vi "Data Queue manager.vi"(5 "queue size":i32, 7 "Action":T1=enum."Enqueue", 8 "error in":errorcluster, 11 "Buffer":sgl[](array[numeric])) -> (0 "error out":errorcluster, 2 "Empty?":bool, 3 "data out":sgl[](array[numeric]))   [LabVIEW 2018]
uses:
  Controls/Queue Manager Actions.ctl
  Controls/QueueNames.ctl
  Controls/MessagePacket.ctl
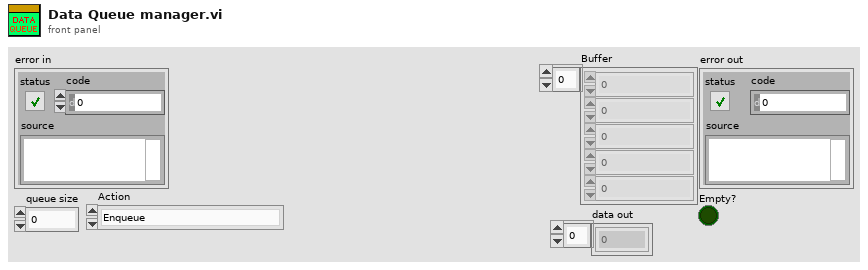
[diagram p1: front panel]
types:
  T1 = typedef "Queue Manager Actions.ctl" = enum16{"Init", "Enqueue", "Enqueue All", "Preview Queue", "Dequeue", "Get Status", "Flush Queue", "Flush All Queues", "Release All Queues", "Release Queue", "Enqueue at Opposite End"}
  T2 = typedef "MessagePacket.ctl" = cluster{"Message":string, "Parameter":variant}
  T3 = typedef "QueueNames.ctl" = enum16{"Main GUI", "Main Scan Processor", "Main Processing", "Main Saving", "Main Display", "Main Table Stage GUI", "Main Table Stage Proc.", "Scan Engine", "Vibratome GUI", "Vibratome Processor", "Slice Engine"}
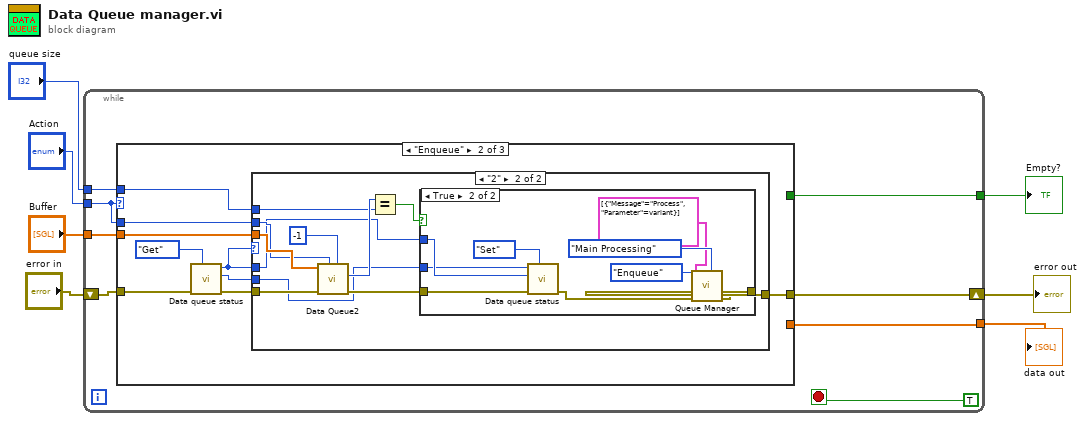
[diagram p0: block diagram]
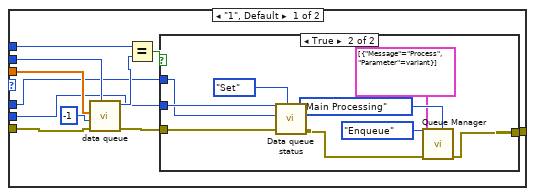
[diagram p3: hidden frame]
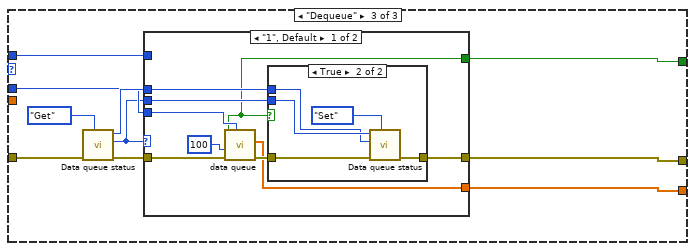
[diagram p6: hidden frame]
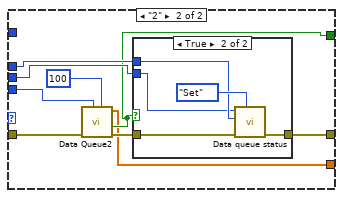
[diagram p8: hidden frame]
diagram:
  n1 = while {
    tunnel: "Buffer" -> [w15]
    tunnel: "Action" -> [w14]
    tunnel: "queue size" -> [w12]
    shift-right: [w11] -> w3
    shift-left: "error in" -> [w13]
    tunnel: [w9] -> w2
    tunnel: [w8] -> w1
    stop <- TRUE stop-if-true
    n2 = case shown="\"Enqueue\"" w14 {
      tunnel: w15 -> [_ w25 _]
      tunnel: w13 -> [w16 w22 w74]
      tunnel: w14 -> [_ w24 w73]
      tunnel: w12 -> [_ w20 w72]
      tunnel: [w16 w17 w71] -> w11
      tunnel: [_ _ w69] -> w9
      tunnel: [_ _ w68] -> w8
      frame "Init", Default {
      }
      frame "Enqueue" {
        n3 = call "Data queue status.vi"("action"=enum16{"Init", "Get", "Set"}."Get", "error in"=w22) -> ("error out"=w21:errorcluster, "dequeue channel"=w18:enum16{"1", "2"}, "enqueue channel"=w19:enum16{"1", "2"})  [unwired: 7 in]
        n4 = case shown="\"2\"" w19 {
          tunnel: w25 -> [w32 w56]
          tunnel: w24 -> [w31 w55]
          tunnel: w21 -> [w35 w57]
          tunnel: w20 -> [w29 w52]
          tunnel: w19 -> [w27 w49]
          tunnel: w18 -> [w28 w48]
          tunnel: [w26 w47] -> w17
          frame "1", Default {
            n5 = call "data queue.vi"("Action"=w31, "error in (no error)"=w35, "timeout in ms (-1)"=-1, "data in"=w32) -> ("error out"=w34:errorcluster, "# elements in queue"=w30:i32)  [unwired: 4 in, 2 out]
            n6 = Equal?(x=w29, y=w30) -> (x = y?=w36:bool)
            n7 = case shown="True" w36 {
              tunnel: [w37 w39] -> w26
              tunnel: w34 -> [w37 w45]
              tunnel: w28 -> [_ w44]
              tunnel: w27 -> [_ w43]
              frame False {
              }
              frame True {
                n8 = call "Data queue status.vi"("action"=enum16{"Init", "Get", "Set"}."Set", "error in"=w45, "dequeue channel"=w43, "enqueue channel"=w44) -> ("error out"=w40:errorcluster)  [unwired: 5 in, 2 out]
                n9 = call "Queue Manager.vi"("Queue Name"=QueueNames."Main Processing", "Action"=Queue_Manager_Actions."Enqueue", "Error In"=w40, "Message Packet Array"=T2[] [{"Message"="Process", "Parameter"=variant}]) -> ("Error Out"=w39:errorcluster)  [unwired: 3 in, 4 out]
              }
            }
          }
          frame "2" {
            n10 = call "Data Queue2.vi"("timeout in ms (-1)"=-1, "Action"=w55, "error in (no error)"=w57, "data in"=w56) -> ("error out"=w50:errorcluster, "# elements in queue"=w53:i32)  [unwired: 4 in, 2 out]
            n11 = Equal?(x=w53, y=w52) -> (x = y?=w51:bool)
            n12 = case shown="True" w51 {
              tunnel: w50 -> [w58 w66]
              tunnel: w49 -> [_ w65]
              tunnel: w48 -> [_ w64]
              tunnel: [w58 w60] -> w47
              frame False {
              }
              frame True {
                n13 = call "Data queue status.vi"("action"=enum16{"Init", "Get", "Set"}."Set", "error in"=w66, "dequeue channel"=w65, "enqueue channel"=w64) -> ("error out"=w61:errorcluster)  [unwired: 5 in, 2 out]
                n14 = call "Queue Manager.vi"("Queue Name"=QueueNames."Main Processing", "Action"=Queue_Manager_Actions."Enqueue", "Error In"=w61, "Message Packet Array"=T2[] [{"Message"="Process", "Parameter"=variant}]) -> ("Error Out"=w60:errorcluster)  [unwired: 3 in, 4 out]
              }
            }
          }
        }
      }
      frame "Dequeue" {
        n15 = call "Data queue status.vi"("action"=enum16{"Init", "Get", "Set"}."Get", "error in"=w74) -> ("error out"=w76:errorcluster, "dequeue channel"=w70:enum16{"1", "2"}, "enqueue channel"=w75:enum16{"1", "2"})  [unwired: 7 in]
        n16 = case shown="\"1\", Default" w70 {
          tunnel: w73 -> [w83 w100]
          tunnel: w76 -> [w86 w101]
          tunnel: w72 -> [_ _]
          tunnel: w75 -> [w81 w97]
          tunnel: w70 -> [w82 w96]
          tunnel: [w80 w95] -> w71
          tunnel: [w79 w94] -> w69
          tunnel: [w78 w93] -> w68
          frame "1", Default {
            n17 = call "data queue.vi"("Action"=w83, "error in (no error)"=w86, "timeout in ms (-1)"=100) -> ("error out"=w85:errorcluster, "data out"=w78:sgl[], "Empty?"=w79:bool)  [unwired: 5 in, 1 out]
            n18 = case shown="True" w79 {
              tunnel: [w87 w91] -> w80
              tunnel: w85 -> [w87 w90]
              tunnel: w82 -> [_ w89]
              tunnel: w81 -> [_ w88]
              frame False {
              }
              frame True {
                n19 = call "Data queue status.vi"("action"=enum16{"Init", "Get", "Set"}."Set", "error in"=w90, "dequeue channel"=w88, "enqueue channel"=w89) -> ("error out"=w91:errorcluster)  [unwired: 5 in, 2 out]
              }
            }
          }
          frame "2" {
            n20 = call "Data Queue2.vi"("timeout in ms (-1)"=100, "Action"=w100, "error in (no error)"=w101) -> ("error out"=w98:errorcluster, "Empty?"=w94:bool, "data out"=w93:sgl[])  [unwired: 5 in, 1 out]
            n21 = case shown="True" w94 {
              tunnel: w98 -> [w102 w106]
              tunnel: w97 -> [_ w105]
              tunnel: w96 -> [_ w104]
              tunnel: [w102 w103] -> w95
              frame False {
              }
              frame True {
                n22 = call "Data queue status.vi"("action"=enum16{"Init", "Get", "Set"}."Set", "error in"=w106, "dequeue channel"=w105, "enqueue channel"=w104) -> ("error out"=w103:errorcluster)  [unwired: 5 in, 2 out]
              }
            }
          }
        }
      }
    }
  }
  "error out" <- w3
  "Empty?" <- w2
  "data out" <- w1
